vi "triquimejorado2.vi"() -> ()   [LabVIEW 2021]
panel:
  out "ocupado 9":bool
  out "ocupado 8":bool
  out "ocupado 7":bool
  out "ocupado 6":bool
  out "ocupado 5":bool
  out "ocupado 4":bool
  out "ocupado 3":bool
  out "ocupado 2":bool
  out "ocupado1":bool
  out "appended array":u16[][](array[numeric])
  in  "OK Button":bool
  in  "x":bool
  in  "Ring 9":u16(ring)
  in  "Ring 8":u16(ring)
  in  "Ring 6":u16(ring)
  in  "Ring 5":u16(ring)
  in  "Ring 7":u16(ring)
  in  "Ring 4":u16(ring)
  in  "Ring 3":u16(ring)
  in  "Ring 2":u16(ring)
  in  "Ring":u16(ring)
  # "TRIQUI"
  # "TURNO"
  # "0"
  # "OCUPACION"
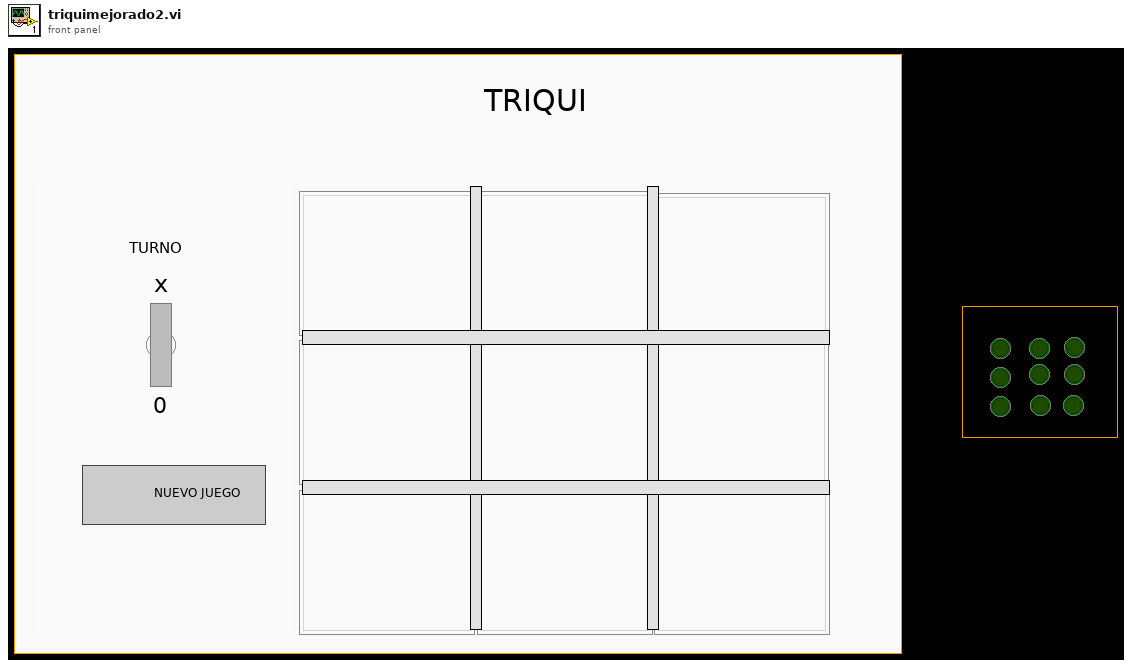
[diagram p1: front panel]
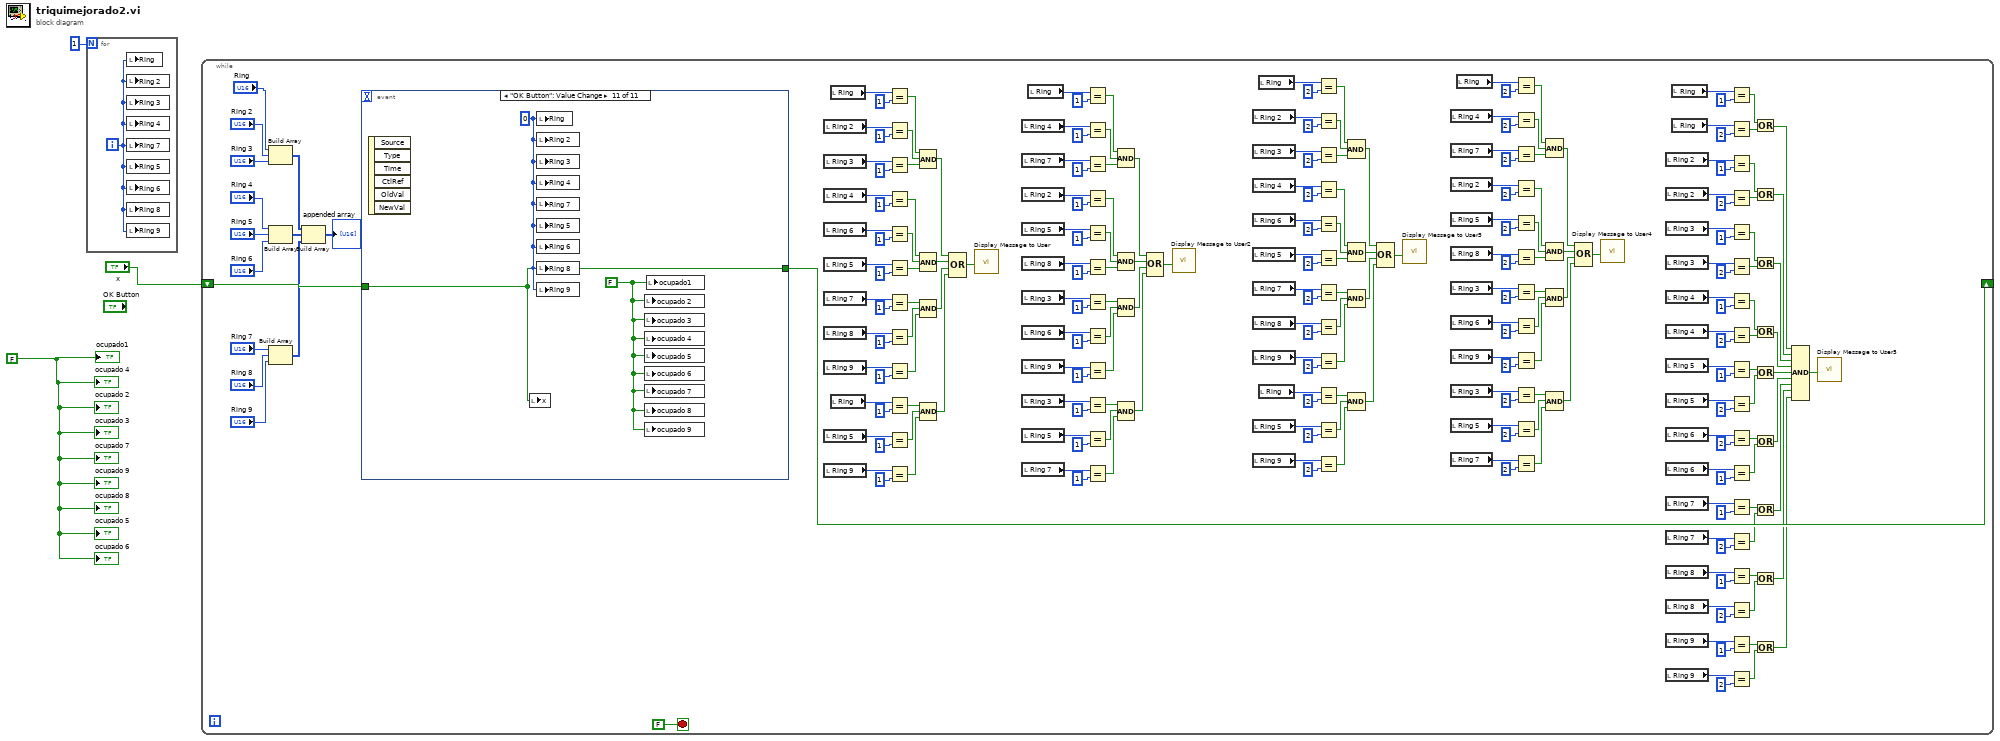
[diagram p0: block diagram]
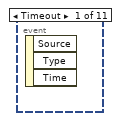
[diagram p2: hidden frame]
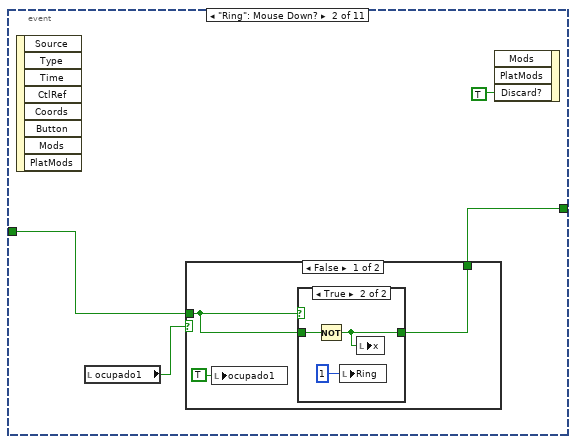
[diagram p3: hidden frame]
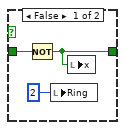
[diagram p4: hidden frame]
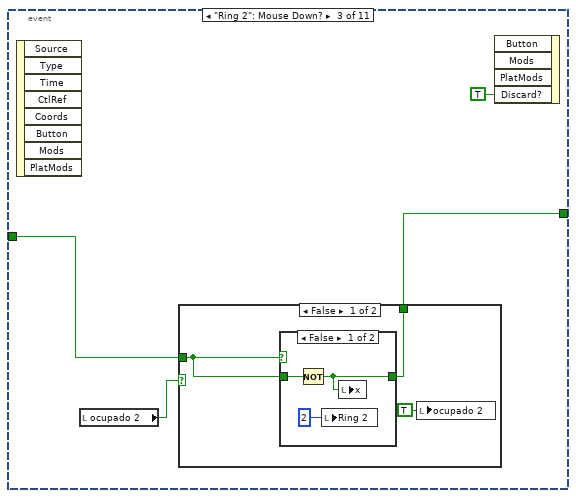
[diagram p6: hidden frame]
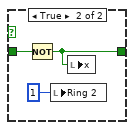
[diagram p7: hidden frame]
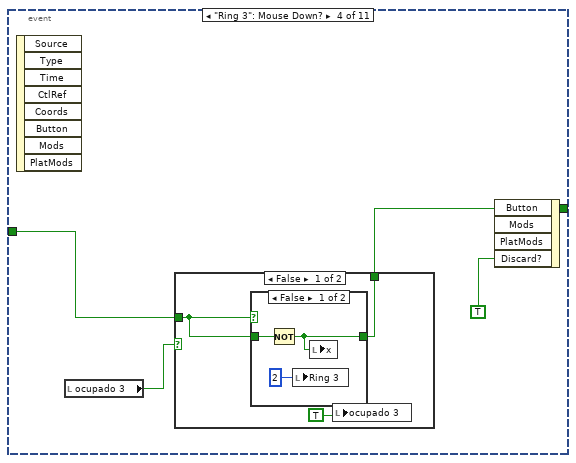
[diagram p9: hidden frame]
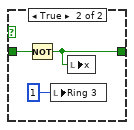
[diagram p10: hidden frame]
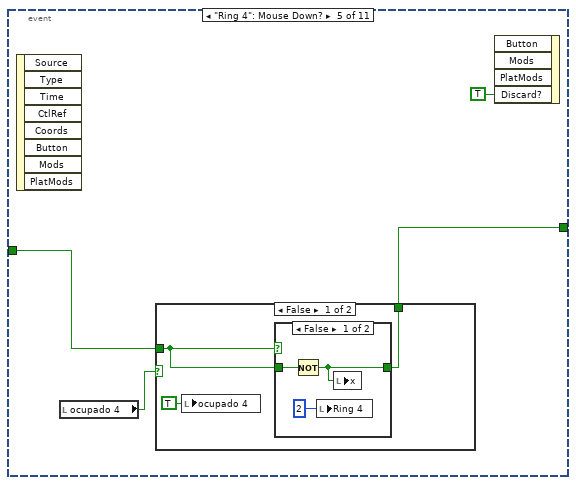
[diagram p12: hidden frame]
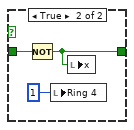
[diagram p13: hidden frame]
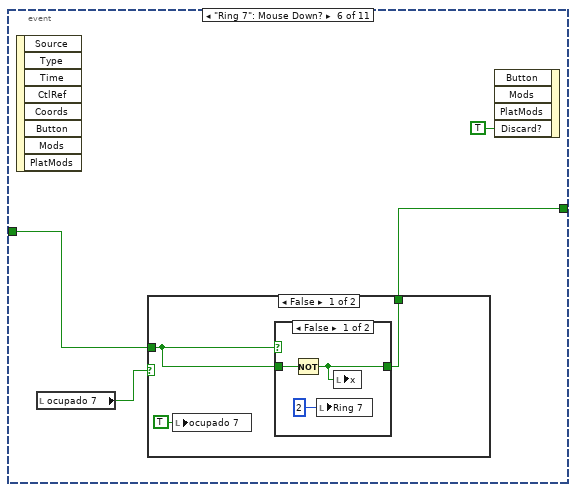
[diagram p15: hidden frame]
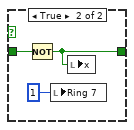
[diagram p16: hidden frame]
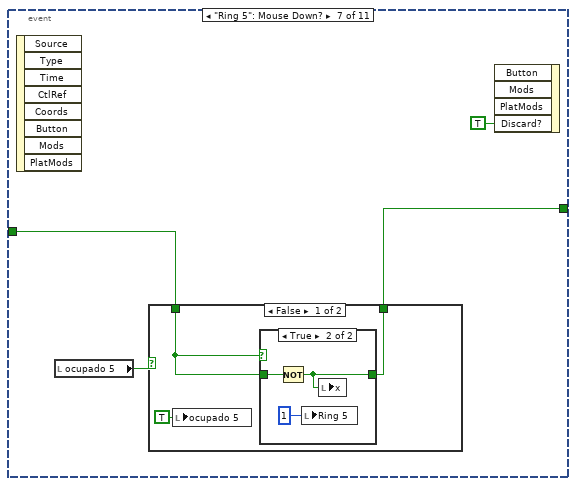
[diagram p18: hidden frame]
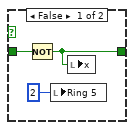
[diagram p19: hidden frame]
diagram:
  w1 = FALSE ("ocupado1")
  n1 = for {
    N: 1 -> [_]
    i -> [w4]
    n2 = local write "Ring"(w4) -> ()
    n3 = local write "Ring 2"(w4) -> ()
    n4 = local write "Ring 3"(w4) -> ()
    n5 = local write "Ring 4"(w4) -> ()
    n6 = local write "Ring 7"(w4) -> ()
    n7 = local write "Ring 5"(w4) -> ()
    n8 = local write "Ring 6"(w4) -> ()
    n9 = local write "Ring 8"(w4) -> ()
    n10 = local write "Ring 9"(w4) -> ()
  }
  n11 = while {
    shift-right: [w248] -> _
    shift-left: "x" -> [w247]
    stop <- FALSE stop-if-true
    n12 = Build Array("Ring", "Ring 2", "Ring 3") -> (w76:u16[])
    n13 = Build Array("Ring 4", "Ring 5", "Ring 6") -> (w75:u16[])
    n14 = Build Array("Ring 7", "Ring 8", "Ring 9") -> (w77:u16[])
    n15 = Build Array(w76, w75, w77) -> (→"appended array":u16[][])
    n16 = event shown="[10] \"OK Button\": Value Change" {
      selector: _ -> [_ _ _ _ _ _ _ _ _ _ _]
      dyn-events: _ -> [_ _ _ _ _ _ _ _ _ _ _]
      timeout: _ -> [_ _ _ _ _ _ _ _ _ _ _]
      tunnel: [_ w250 w264 w278 w292 w306 w320 w334 w348 w362 w376] -> w248
      tunnel: w247 -> [_ w251 w265 w279 w293 w307 w321 w335 w349 w363 w376]
      event Timeout {
        n17 = event-data() -> ()  [unwired: 1 in, 3 out]
      }
      event "Ring": Mouse Down? {
        n18 = event-data() -> ()  [unwired: 1 in, 8 out]
        n19 = local read "ocupado1"() -> (w249:bool)
        n20 = case shown="False" w249 {
          tunnel: w251 -> [w255 w262]
          tunnel: [w254 w262] -> w250
          frame False {
            n21 = local write "ocupado1"(TRUE ("ocupado1")) -> ()
            n22 = case shown="True" w255 {
              tunnel: [w257 w260] -> w254
              tunnel: w255 -> [w256 w259]
              frame False {
                n23 = Not(x=w256) -> (.not. x?=w257:bool)
                n24 = local write "Ring"(u16 2 ("Ring")) -> ()
                n25 = local write "x"(w257) -> ()
              }
              frame True {
                n26 = Not(x=w259) -> (.not. x?=w260:bool)
                n27 = local write "Ring"(u16 1 ("Ring")) -> ()
                n28 = local write "x"(w260) -> ()
              }
            }
          }
          frame True {
          }
        }
        n29 = event-data("Discard?"=TRUE) -> ()  [unwired: 3 in, 1 out]
      }
      event "Ring 2": Mouse Down? {
        n30 = event-data() -> ()  [unwired: 1 in, 8 out]
        n31 = local read "ocupado 2"() -> (w263:bool)
        n32 = case shown="False" w263 {
          tunnel: w265 -> [w269 w276]
          tunnel: [w268 w276] -> w264
          frame False {
            n33 = case shown="False" w269 {
              tunnel: w269 -> [w271 w274]
              tunnel: [w270 w273] -> w268
              frame False {
                n34 = Not(x=w271) -> (.not. x?=w270:bool)
                n35 = local write "Ring 2"(u16 2 ("Ring 2")) -> ()
                n36 = local write "x"(w270) -> ()
              }
              frame True {
                n37 = Not(x=w274) -> (.not. x?=w273:bool)
                n38 = local write "Ring 2"(u16 1 ("Ring 2")) -> ()
                n39 = local write "x"(w273) -> ()
              }
            }
            n40 = local write "ocupado 2"(TRUE ("ocupado 2")) -> ()
          }
          frame True {
          }
        }
        n41 = event-data("Discard?"=TRUE) -> ()  [unwired: 4 in, 1 out]
      }
      event "Ring 3": Mouse Down? {
        n42 = event-data() -> ()  [unwired: 1 in, 8 out]
        n43 = local read "ocupado 3"() -> (w277:bool)
        n44 = case shown="False" w277 {
          tunnel: w279 -> [w283 w290]
          tunnel: [w282 w290] -> w278
          frame False {
            n45 = case shown="False" w283 {
              tunnel: w283 -> [w285 w288]
              tunnel: [w284 w287] -> w282
              frame False {
                n46 = Not(x=w285) -> (.not. x?=w284:bool)
                n47 = local write "Ring 3"(u16 2 ("Ring 2")) -> ()
                n48 = local write "x"(w284) -> ()
              }
              frame True {
                n49 = Not(x=w288) -> (.not. x?=w287:bool)
                n50 = local write "Ring 3"(u16 1 ("Ring 2")) -> ()
                n51 = local write "x"(w287) -> ()
              }
            }
            n52 = local write "ocupado 3"(TRUE ("ocupado 3")) -> ()
          }
          frame True {
          }
        }
        n53 = event-data("Discard?"=TRUE) -> ()  [unwired: 4 in, 1 out]
      }
      event "Ring 4": Mouse Down? {
        n54 = event-data() -> ()  [unwired: 1 in, 8 out]
        n55 = local read "ocupado 4"() -> (w291:bool)
        n56 = case shown="False" w291 {
          tunnel: w293 -> [w297 w304]
          tunnel: [w296 w304] -> w292
          frame False {
            n57 = local write "ocupado 4"(TRUE ("ocupado 4")) -> ()
            n58 = case shown="False" w297 {
              tunnel: w297 -> [w299 w302]
              tunnel: [w298 w301] -> w296
              frame False {
                n59 = Not(x=w299) -> (.not. x?=w298:bool)
                n60 = local write "Ring 4"(u16 2 ("Ring 2")) -> ()
                n61 = local write "x"(w298) -> ()
              }
              frame True {
                n62 = Not(x=w302) -> (.not. x?=w301:bool)
                n63 = local write "Ring 4"(u16 1 ("Ring 2")) -> ()
                n64 = local write "x"(w301) -> ()
              }
            }
          }
          frame True {
          }
        }
        n65 = event-data("Discard?"=TRUE) -> ()  [unwired: 4 in, 1 out]
      }
      event "Ring 7": Mouse Down? {
        n66 = event-data() -> ()  [unwired: 1 in, 8 out]
        n67 = local read "ocupado 7"() -> (w305:bool)
        n68 = case shown="False" w305 {
          tunnel: w307 -> [w311 w318]
          tunnel: [w310 w318] -> w306
          frame False {
            n69 = local write "ocupado 7"(TRUE ("ocupado 7")) -> ()
            n70 = case shown="False" w311 {
              tunnel: w311 -> [w313 w316]
              tunnel: [w312 w315] -> w310
              frame False {
                n71 = Not(x=w313) -> (.not. x?=w312:bool)
                n72 = local write "Ring 7"(u16 2 ("Ring 2")) -> ()
                n73 = local write "x"(w312) -> ()
              }
              frame True {
                n74 = Not(x=w316) -> (.not. x?=w315:bool)
                n75 = local write "Ring 7"(u16 1 ("Ring 2")) -> ()
                n76 = local write "x"(w315) -> ()
              }
            }
          }
          frame True {
          }
        }
        n77 = event-data("Discard?"=TRUE) -> ()  [unwired: 4 in, 1 out]
      }
      event "Ring 5": Mouse Down? {
        n78 = event-data() -> ()  [unwired: 1 in, 8 out]
        n79 = local read "ocupado 5"() -> (w319:bool)
        n80 = case shown="False" w319 {
          tunnel: w321 -> [w325 w332]
          tunnel: [w324 w332] -> w320
          frame False {
            n81 = local write "ocupado 5"(TRUE ("ocupado 5")) -> ()
            n82 = case shown="True" w325 {
              tunnel: w325 -> [w327 w330]
              tunnel: [w326 w329] -> w324
              frame False {
                n83 = Not(x=w327) -> (.not. x?=w326:bool)
                n84 = local write "Ring 5"(u16 2 ("Ring 2")) -> ()
                n85 = local write "x"(w326) -> ()
              }
              frame True {
                n86 = Not(x=w330) -> (.not. x?=w329:bool)
                n87 = local write "Ring 5"(u16 1 ("Ring 2")) -> ()
                n88 = local write "x"(w329) -> ()
              }
            }
          }
          frame True {
          }
        }
        n89 = event-data("Discard?"=TRUE) -> ()  [unwired: 4 in, 1 out]
      }
      event "Ring 6": Mouse Down? {
        n90 = event-data() -> ()  [unwired: 1 in, 8 out]
        n91 = local read "ocupado 6"() -> (w333:bool)
        n92 = case shown="True" w333 {
          tunnel: w335 -> [w339 w346]
          tunnel: [w338 w346] -> w334
          frame False {
            n93 = local write "ocupado 6"(TRUE ("ocupado 6")) -> ()
            n94 = case shown="False" w339 {
              tunnel: w339 -> [w341 w344]
              tunnel: [w340 w343] -> w338
              frame False {
                n95 = Not(x=w341) -> (.not. x?=w340:bool)
                n96 = local write "Ring 6"(u16 2 ("Ring 2")) -> ()
                n97 = local write "x"(w340) -> ()
              }
              frame True {
                n98 = Not(x=w344) -> (.not. x?=w343:bool)
                n99 = local write "Ring 6"(u16 1 ("Ring 2")) -> ()
                n100 = local write "x"(w343) -> ()
              }
            }
          }
          frame True {
          }
        }
        n101 = event-data("Discard?"=TRUE) -> ()  [unwired: 4 in, 1 out]
      }
      event "Ring 8": Mouse Down? {
        n102 = event-data() -> ()  [unwired: 1 in, 8 out]
        n103 = local read "ocupado 8"() -> (w347:bool)
        n104 = case shown="False" w347 {
          tunnel: w349 -> [w353 w360]
          tunnel: [w352 w360] -> w348
          frame False {
            n105 = local write "ocupado 8"(TRUE ("ocupado 8")) -> ()
            n106 = case shown="False" w353 {
              tunnel: w353 -> [w355 w358]
              tunnel: [w354 w357] -> w352
              frame False {
                n107 = Not(x=w355) -> (.not. x?=w354:bool)
                n108 = local write "Ring 8"(u16 2 ("Ring 2")) -> ()
                n109 = local write "x"(w354) -> ()
              }
              frame True {
                n110 = Not(x=w358) -> (.not. x?=w357:bool)
                n111 = local write "Ring 8"(u16 1 ("Ring 2")) -> ()
                n112 = local write "x"(w357) -> ()
              }
            }
          }
          frame True {
          }
        }
        n113 = event-data("Discard?"=TRUE) -> ()  [unwired: 4 in, 1 out]
      }
      event "Ring 9": Mouse Down? {
        n114 = event-data() -> ()  [unwired: 1 in, 8 out]
        n115 = local read "ocupado 9"() -> (w361:bool)
        n116 = case shown="False" w361 {
          tunnel: w363 -> [w367 w374]
          tunnel: [w366 w374] -> w362
          frame False {
            n117 = local write "ocupado 9"(TRUE ("ocupado 9")) -> ()
            n118 = case shown="False" w367 {
              tunnel: w367 -> [w369 w372]
              tunnel: [w368 w371] -> w366
              frame False {
                n119 = Not(x=w369) -> (.not. x?=w368:bool)
                n120 = local write "Ring 9"(u16 2 ("Ring 2")) -> ()
                n121 = local write "x"(w368) -> ()
              }
              frame True {
                n122 = Not(x=w372) -> (.not. x?=w371:bool)
                n123 = local write "Ring 9"(u16 1 ("Ring 2")) -> ()
                n124 = local write "x"(w371) -> ()
              }
            }
          }
          frame True {
          }
        }
        n125 = event-data("Discard?"=TRUE) -> ()  [unwired: 4 in, 1 out]
      }
      event "OK Button": Value Change {
        w375 = FALSE ("ocupado1")
        w377 = u16 0 ("Ring")
        n126 = event-data() -> ()  [unwired: 1 in, 6 out]
        n127 = local write "x"(w376) -> ()
        n128 = local write "Ring"(w377) -> ()
        n129 = local write "Ring 2"(w377) -> ()
        n130 = local write "Ring 3"(w377) -> ()
        n131 = local write "Ring 4"(w377) -> ()
        n132 = local write "Ring 7"(w377) -> ()
        n133 = local write "Ring 5"(w377) -> ()
        n134 = local write "Ring 6"(w377) -> ()
        n135 = local write "Ring 8"(w377) -> ()
        n136 = local write "Ring 9"(w377) -> ()
        n137 = local write "ocupado 2"(w375) -> ()
        n138 = local write "ocupado 3"(w375) -> ()
        n139 = local write "ocupado 4"(w375) -> ()
        n140 = local write "ocupado 5"(w375) -> ()
        n141 = local write "ocupado 6"(w375) -> ()
        n142 = local write "ocupado 7"(w375) -> ()
        n143 = local write "ocupado 8"(w375) -> ()
        n144 = local write "ocupado 9"(w375) -> ()
        n145 = local write "ocupado1"(w375) -> ()
      }
    }
    n146 = local read "Ring 2"() -> (w244:u16)
    n147 = local read "Ring 3"() -> (w242:u16)
    n148 = local read "Ring 4"() -> (w231:u16)
    n149 = local read "Ring 6"() -> (w230:u16)
    n150 = local read "Ring 5"() -> (w229:u16)
    n151 = local read "Ring 7"() -> (w222:u16)
    n152 = local read "Ring 8"() -> (w221:u16)
    n153 = local read "Ring 9"() -> (w220:u16)
    n154 = local read "Ring 5"() -> (w214:u16)
    n155 = local read "Ring 9"() -> (w215:u16)
    n156 = local read "Ring"() -> (w246:u16)
    n157 = local read "Ring"() -> (w213:u16)
    n158 = Equal?(x=w246, y=u16 1) -> (x = y?=w240:bool)
    n159 = Equal?(x=w244, y=u16 1) -> (x = y?=w239:bool)
    n160 = Equal?(x=w242, y=u16 1) -> (x = y?=w238:bool)
    n161 = Equal?(x=w231, y=u16 1) -> (x = y?=w235:bool)
    n162 = Equal?(x=w230, y=u16 1) -> (x = y?=w236:bool)
    n163 = Equal?(x=w229, y=u16 1) -> (x = y?=w237:bool)
    n164 = Equal?(x=w222, y=u16 1) -> (x = y?=w225:bool)
    n165 = Equal?(x=w221, y=u16 1) -> (x = y?=w224:bool)
    n166 = Equal?(x=w220, y=u16 1) -> (x = y?=w223:bool)
    n167 = Equal?(x=w213, y=u16 1) -> (x = y?=w210:bool)
    n168 = Equal?(x=w214, y=u16 1) -> (x = y?=w211:bool)
    n169 = Equal?(x=w215, y=u16 1) -> (x = y?=w212:bool)
    n170 = Compound Arithmetic op=AND(w240, w239, w238) -> (w219:bool)
    n171 = Compound Arithmetic op=AND(w235, w236, w237) -> (w218:bool)
    n172 = Compound Arithmetic op=AND(w225, w224, w223) -> (w217:bool)
    n173 = Compound Arithmetic op=AND(w210, w211, w212) -> (w206:bool)
    n174 = Compound Arithmetic op=OR(w219, w218, w217, w206) -> (w216:bool)
    n175 = call "Display Message to User"("Enable"=w216) -> ()  [unwired: 9 in, 2 out]
    n176 = local read "Ring 4"() -> (w167:u16)
    n177 = local read "Ring 7"() -> (w169:u16)
    n178 = local read "Ring 2"() -> (w180:u16)
    n179 = local read "Ring 5"() -> (w181:u16)
    n180 = local read "Ring 8"() -> (w182:u16)
    n181 = local read "Ring 3"() -> (w189:u16)
    n182 = local read "Ring 6"() -> (w190:u16)
    n183 = local read "Ring 9"() -> (w191:u16)
    n184 = local read "Ring 3"() -> (w198:u16)
    n185 = local read "Ring 5"() -> (w197:u16)
    n186 = local read "Ring 7"() -> (w196:u16)
    n187 = local read "Ring"() -> (w165:u16)
    n188 = Equal?(x=w165, y=u16 1) -> (x = y?=w171:bool)
    n189 = Equal?(x=w167, y=u16 1) -> (x = y?=w172:bool)
    n190 = Equal?(x=w169, y=u16 1) -> (x = y?=w173:bool)
    n191 = Equal?(x=w180, y=u16 1) -> (x = y?=w176:bool)
    n192 = Equal?(x=w181, y=u16 1) -> (x = y?=w175:bool)
    n193 = Equal?(x=w182, y=u16 1) -> (x = y?=w174:bool)
    n194 = Equal?(x=w189, y=u16 1) -> (x = y?=w186:bool)
    n195 = Equal?(x=w190, y=u16 1) -> (x = y?=w187:bool)
    n196 = Equal?(x=w191, y=u16 1) -> (x = y?=w188:bool)
    n197 = Equal?(x=w198, y=u16 1) -> (x = y?=w201:bool)
    n198 = Equal?(x=w197, y=u16 1) -> (x = y?=w200:bool)
    n199 = Equal?(x=w196, y=u16 1) -> (x = y?=w199:bool)
    n200 = Compound Arithmetic op=AND(w171, w172, w173) -> (w192:bool)
    n201 = Compound Arithmetic op=AND(w176, w175, w174) -> (w193:bool)
    n202 = Compound Arithmetic op=AND(w186, w187, w188) -> (w194:bool)
    n203 = Compound Arithmetic op=AND(w201, w200, w199) -> (w205:bool)
    n204 = Compound Arithmetic op=OR(w192, w193, w194, w205) -> (w195:bool)
    n205 = call "Display Message to User2"("Enable"=w195) -> ()  [unwired: 9 in, 2 out]
    n206 = local read "Ring 2"() -> (w85:u16)
    n207 = local read "Ring 3"() -> (w87:u16)
    n208 = local read "Ring 4"() -> (w98:u16)
    n209 = local read "Ring 6"() -> (w99:u16)
    n210 = local read "Ring 5"() -> (w100:u16)
    n211 = local read "Ring 7"() -> (w107:u16)
    n212 = local read "Ring 8"() -> (w108:u16)
    n213 = local read "Ring 9"() -> (w109:u16)
    n214 = local read "Ring 5"() -> (w115:u16)
    n215 = local read "Ring 9"() -> (w114:u16)
    n216 = local read "Ring"() -> (w83:u16)
    n217 = local read "Ring"() -> (w116:u16)
    n218 = Equal?(x=w83, y=u16 2) -> (x = y?=w89:bool)
    n219 = Equal?(x=w85, y=u16 2) -> (x = y?=w90:bool)
    n220 = Equal?(x=w87, y=u16 2) -> (x = y?=w91:bool)
    n221 = Equal?(x=w98, y=u16 2) -> (x = y?=w94:bool)
    n222 = Equal?(x=w99, y=u16 2) -> (x = y?=w93:bool)
    n223 = Equal?(x=w100, y=u16 2) -> (x = y?=w92:bool)
    n224 = Equal?(x=w107, y=u16 2) -> (x = y?=w104:bool)
    n225 = Equal?(x=w108, y=u16 2) -> (x = y?=w105:bool)
    n226 = Equal?(x=w109, y=u16 2) -> (x = y?=w106:bool)
    n227 = Equal?(x=w116, y=u16 2) -> (x = y?=w119:bool)
    n228 = Equal?(x=w115, y=u16 2) -> (x = y?=w118:bool)
    n229 = Equal?(x=w114, y=u16 2) -> (x = y?=w117:bool)
    n230 = Compound Arithmetic op=AND(w89, w90, w91) -> (w110:bool)
    n231 = Compound Arithmetic op=AND(w94, w93, w92) -> (w111:bool)
    n232 = Compound Arithmetic op=AND(w104, w105, w106) -> (w112:bool)
    n233 = Compound Arithmetic op=AND(w119, w118, w117) -> (w123:bool)
    n234 = Compound Arithmetic op=OR(w110, w111, w112, w123) -> (w113:bool)
    n235 = call "Display Message to User3"("Enable"=w113) -> ()  [unwired: 9 in, 2 out]
    n236 = local read "Ring 4"() -> (w162:u16)
    n237 = local read "Ring 7"() -> (w160:u16)
    n238 = local read "Ring 2"() -> (w149:u16)
    n239 = local read "Ring 5"() -> (w148:u16)
    n240 = local read "Ring 8"() -> (w147:u16)
    n241 = local read "Ring 3"() -> (w140:u16)
    n242 = local read "Ring 6"() -> (w139:u16)
    n243 = local read "Ring 9"() -> (w138:u16)
    n244 = local read "Ring 3"() -> (w131:u16)
    n245 = local read "Ring 5"() -> (w132:u16)
    n246 = local read "Ring 7"() -> (w133:u16)
    n247 = local read "Ring"() -> (w164:u16)
    n248 = Equal?(x=w164, y=u16 2) -> (x = y?=w158:bool)
    n249 = Equal?(x=w162, y=u16 2) -> (x = y?=w157:bool)
    n250 = Equal?(x=w160, y=u16 2) -> (x = y?=w156:bool)
    n251 = Equal?(x=w149, y=u16 2) -> (x = y?=w153:bool)
    n252 = Equal?(x=w148, y=u16 2) -> (x = y?=w154:bool)
    n253 = Equal?(x=w147, y=u16 2) -> (x = y?=w155:bool)
    n254 = Equal?(x=w140, y=u16 2) -> (x = y?=w143:bool)
    n255 = Equal?(x=w139, y=u16 2) -> (x = y?=w142:bool)
    n256 = Equal?(x=w138, y=u16 2) -> (x = y?=w141:bool)
    n257 = Equal?(x=w131, y=u16 2) -> (x = y?=w128:bool)
    n258 = Equal?(x=w132, y=u16 2) -> (x = y?=w129:bool)
    n259 = Equal?(x=w133, y=u16 2) -> (x = y?=w130:bool)
    n260 = Compound Arithmetic op=AND(w158, w157, w156) -> (w137:bool)
    n261 = Compound Arithmetic op=AND(w153, w154, w155) -> (w136:bool)
    n262 = Compound Arithmetic op=AND(w143, w142, w141) -> (w135:bool)
    n263 = Compound Arithmetic op=AND(w128, w129, w130) -> (w124:bool)
    n264 = Compound Arithmetic op=OR(w137, w136, w135, w124) -> (w134:bool)
    n265 = call "Display Message to User4"("Enable"=w134) -> ()  [unwired: 9 in, 2 out]
    n266 = local read "Ring 2"() -> (w61:u16)
    n267 = local read "Ring 2"() -> (w64:u16)
    n268 = local read "Ring 3"() -> (w60:u16)
    n269 = local read "Ring 3"() -> (w57:u16)
    n270 = local read "Ring 4"() -> (w53:u16)
    n271 = local read "Ring 4"() -> (w56:u16)
    n272 = local read "Ring 5"() -> (w52:u16)
    n273 = local read "Ring 5"() -> (w49:u16)
    n274 = local read "Ring 6"() -> (w48:u16)
    n275 = local read "Ring 6"() -> (w45:u16)
    n276 = local read "Ring 7"() -> (w44:u16)
    n277 = local read "Ring 7"() -> (w41:u16)
    n278 = local read "Ring 8"() -> (w37:u16)
    n279 = local read "Ring 8"() -> (w40:u16)
    n280 = local read "Ring 9"() -> (w36:u16)
    n281 = local read "Ring 9"() -> (w33:u16)
    n282 = local read "Ring"() -> (w68:u16)
    n283 = local read "Ring"() -> (w65:u16)
    n284 = Equal?(x=w68, y=u16 1) -> (x = y?=w32:bool)
    n285 = Equal?(x=w65, y=u16 2) -> (x = y?=w31:bool)
    n286 = Equal?(x=w61, y=u16 1) -> (x = y?=w30:bool)
    n287 = Equal?(x=w64, y=u16 2) -> (x = y?=w29:bool)
    n288 = Equal?(x=w60, y=u16 1) -> (x = y?=w26:bool)
    n289 = Equal?(x=w57, y=u16 2) -> (x = y?=w25:bool)
    n290 = Equal?(x=w53, y=u16 1) -> (x = y?=w24:bool)
    n291 = Equal?(x=w56, y=u16 2) -> (x = y?=w23:bool)
    n292 = Equal?(x=w52, y=u16 1) -> (x = y?=w22:bool)
    n293 = Equal?(x=w49, y=u16 2) -> (x = y?=w21:bool)
    n294 = Equal?(x=w48, y=u16 2) -> (x = y?=w20:bool)
    n295 = Equal?(x=w45, y=u16 1) -> (x = y?=w28:bool)
    n296 = Equal?(x=w44, y=u16 1) -> (x = y?=w19:bool)
    n297 = Equal?(x=w41, y=u16 2) -> (x = y?=w27:bool)
    n298 = Equal?(x=w37, y=u16 1) -> (x = y?=w18:bool)
    n299 = Equal?(x=w40, y=u16 2) -> (x = y?=w17:bool)
    n300 = Equal?(x=w36, y=u16 1) -> (x = y?=w16:bool)
    n301 = Equal?(x=w33, y=u16 2) -> (x = y?=w15:bool)
    n302 = Or(x=w32, y=w31) -> (x .or. y?=w14:bool)
    n303 = Or(x=w30, y=w29) -> (x .or. y?=w13:bool)
    n304 = Or(x=w26, y=w25) -> (x .or. y?=w12:bool)
    n305 = Or(x=w24, y=w23) -> (x .or. y?=w11:bool)
    n306 = Or(x=w22, y=w21) -> (x .or. y?=w10:bool)
    n307 = Or(x=w20, y=w28) -> (x .or. y?=w9:bool)
    n308 = Or(x=w19, y=w27) -> (x .or. y?=w8:bool)
    n309 = Or(x=w18, y=w17) -> (x .or. y?=w7:bool)
    n310 = Or(x=w16, y=w15) -> (x .or. y?=w6:bool)
    n311 = Compound Arithmetic op=AND(w14, w13, w12, w11, w10, w9, w8, w7, w6) -> (w5:bool)
    n312 = call "Display Message to User5"("Enable"=w5) -> ()  [unwired: 9 in, 2 out]
  }
  "ocupado1" <- w1
  "ocupado 2" <- w1
  "ocupado 3" <- w1
  "ocupado 4" <- w1
  "ocupado 5" <- w1
  "ocupado 6" <- w1
  "ocupado 7" <- w1
  "ocupado 8" <- w1
  "ocupado 9" <- w1
